vi "Create.vi"(8 "error in (no error)":errorcluster, 11 "BufferWrites1SamDBL in":refnum<class "BufferWrites1SamDBL.lvclass">) -> (0 "error out":errorcluster, 3 "BufferWrites1SamDBL out":refnum<class "BufferWrites1SamDBL.lvclass">)   [LabVIEW 2024, in "BufferWrites1SamDBL.lvclass"]
uses:
  BufferWrites1SamDBL.lvclass
  BufferWrites1SamDBL.lvclass/BufferWrites1SamDBL.ctl
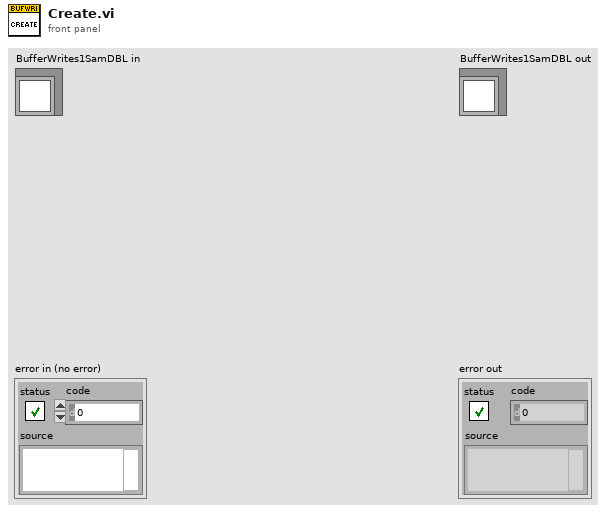
[diagram p1: front panel]
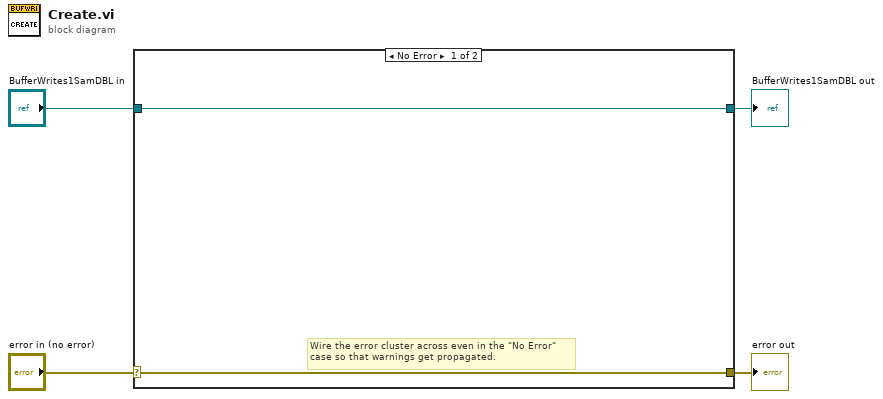
[diagram p0: block diagram]
diagram:
  n1 = case shown="No Error" "error in (no error)" {
    selector: "error in (no error)" -> [w5 w8]
    tunnel: [w5 w8] -> w3
    tunnel: [w6 w7] -> w1
    tunnel: "BufferWrites1SamDBL in" -> [w6 w7]
    frame No Error {
      # "Wire the error cluster across even in the \"No Error\"\ncase so that warnings get propagated."
    }
    frame Error {
    }
  }
  "error out" <- w3
  "BufferWrites1SamDBL out" <- w1
